vi "TestExec.Data Str to DataVariant.vi"(3 "error in":errorcluster, 4 "DataArray":string[](array[string]), 5 "DataStr":string) -> (0 "error out":errorcluster, 2 "Data":variant)   [LabVIEW 2017]
uses:
  Controls/TestExec.Result Cluster, Float.ctl
  Controls/TestExec.Comparison Enum.ctl
  Controls/TestExec.Result Cluster, Int.ctl
  Controls/TestExec.Result Cluster, Bool.ctl
  Controls/TestExec.Result Cluster, Str.ctl
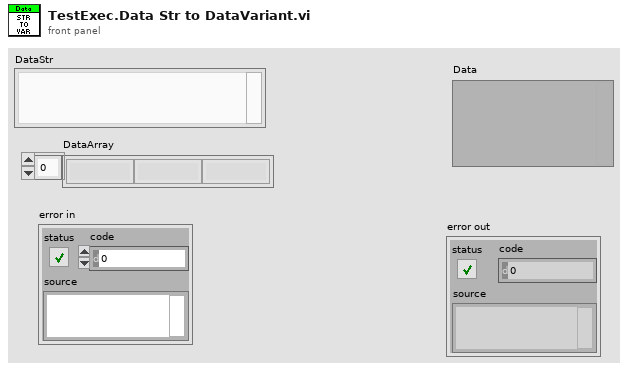
[diagram p1: front panel]
types:
  T1 = typedef "TestExec.Result Cluster, Str.ctl" = cluster{"Desc":string, "Value":string, "Units":string, "LimitName":string, "Comp1":T2, "Lim1":string, "Comp2":T2, "Lim2":string, "FailName":string, "FailCode":dbl, "FailDesc":string, "FailInfo":string}
  T2 = typedef "TestExec.Comparison Enum.ctl" = enum16{"N/A", "EQ", "NEQ", "LT", "LTE", "GT", "GTE"}
  T3 = typedef "TestExec.Result Cluster, Bool.ctl" = cluster{"Desc":string, "Value":bool, "Units":string, "LimitName":string, "Comp1":T2, "Lim1":bool, "FailName":string, "FailCode":dbl, "FailDesc":string, "FailInfo":string}
  T4 = typedef "TestExec.Result Cluster, Int.ctl" = cluster{"Desc":string, "Value":i32, "Units":string, "LimitName":string, "Comp1":T2, "Lim1":i32, "Comp2":T2, "Lim2":i32, "FailName":string, "FailCode":dbl, "FailDesc":string, "FailInfo":string}
  T5 = typedef "TestExec.Result Cluster, Float.ctl" = cluster{"Desc":string, "Value":dbl, "Units":string, "LimitName":string, "Comp1":T2, "Lim1":dbl, "Comp2":T2, "Lim2":dbl, "FailName":string, "FailCode":dbl, "FailDesc":string, "FailInfo":string}
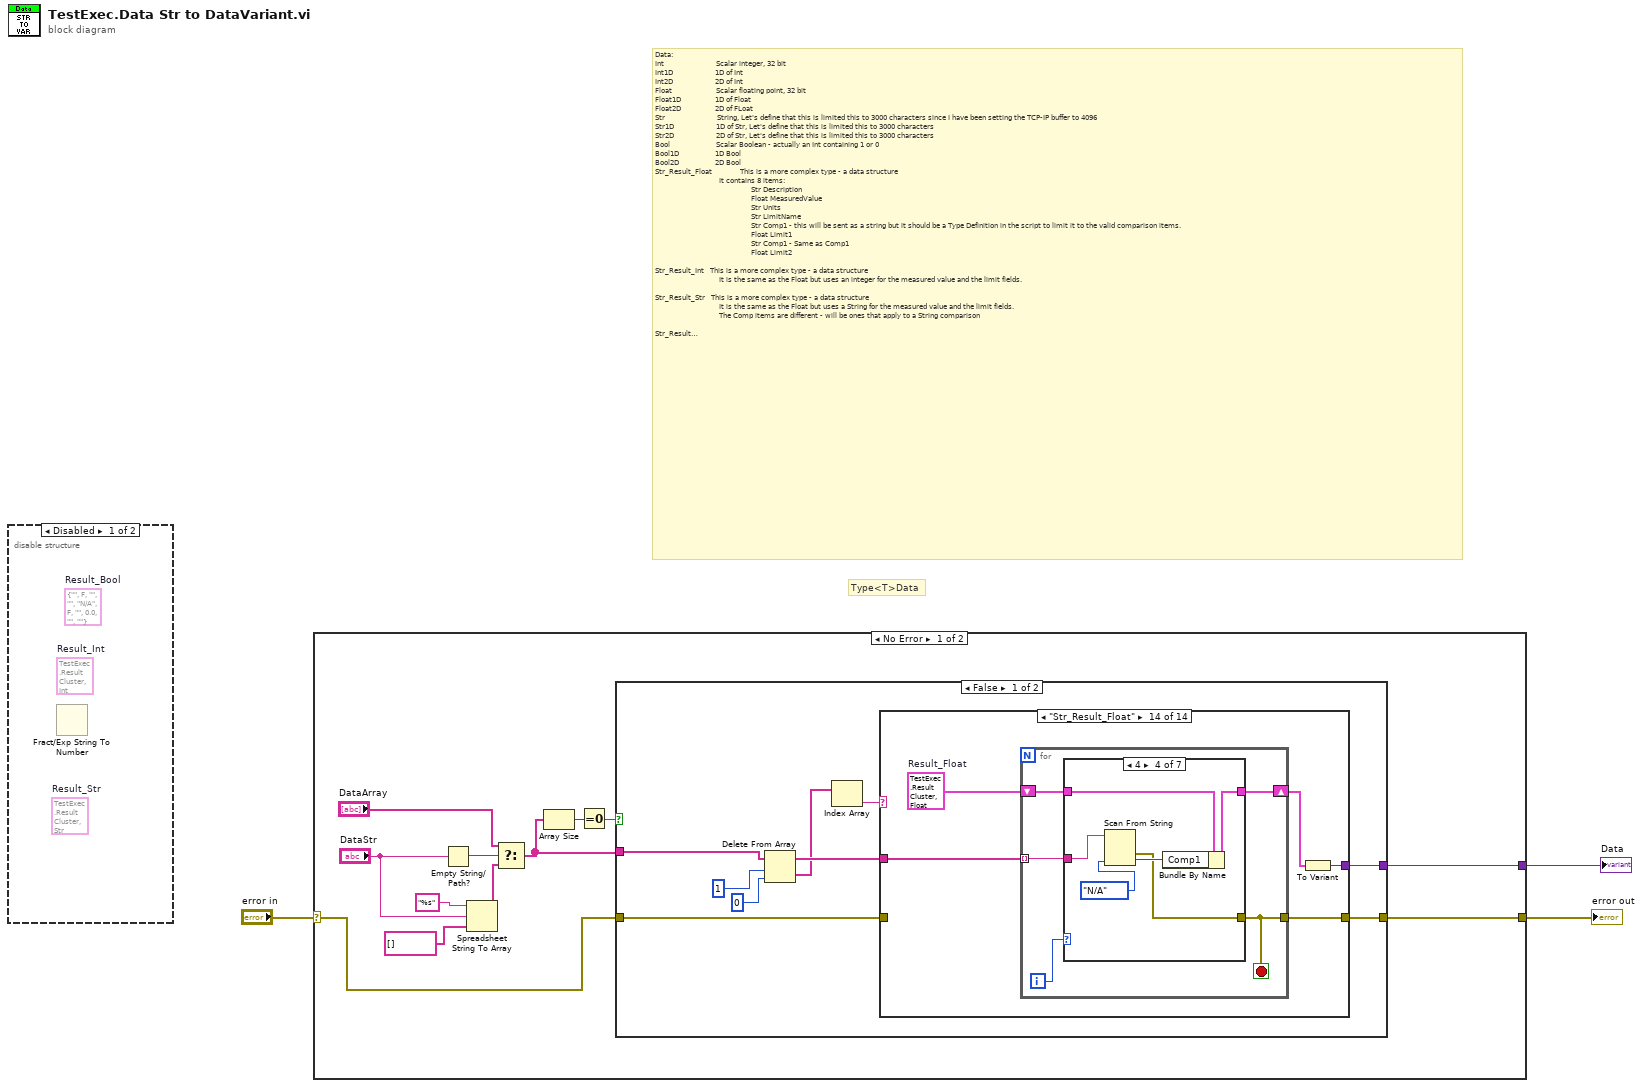
[diagram p0: block diagram]
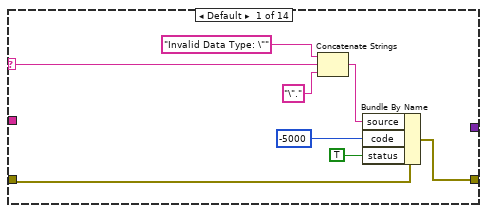
[diagram p3: hidden frame]
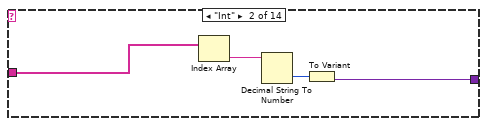
[diagram p4: hidden frame]
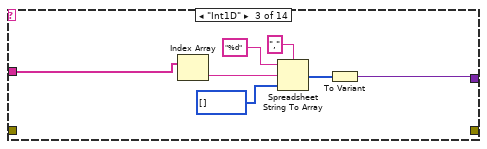
[diagram p5: hidden frame]
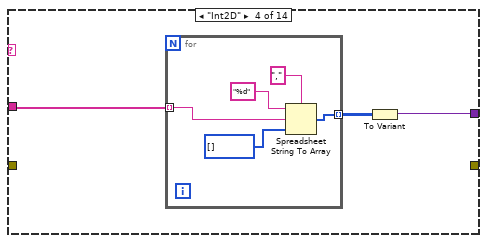
[diagram p6: hidden frame]
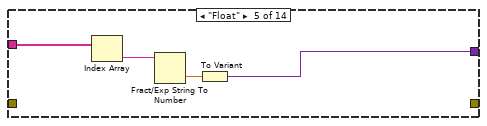
[diagram p7: hidden frame]
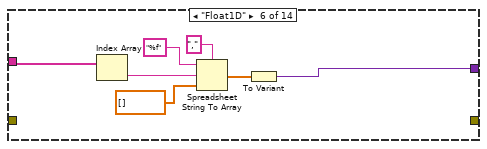
[diagram p8: hidden frame]
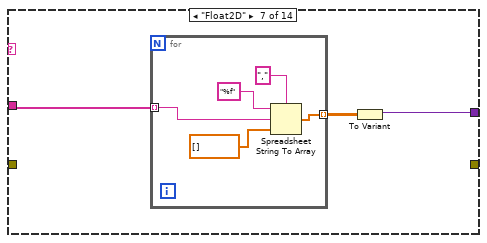
[diagram p9: hidden frame]
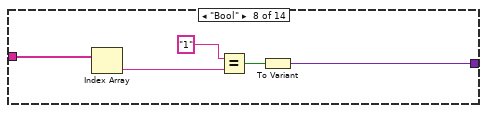
[diagram p10: hidden frame]
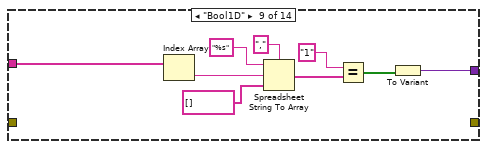
[diagram p11: hidden frame]
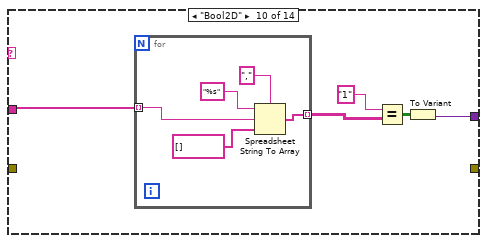
[diagram p12: hidden frame]
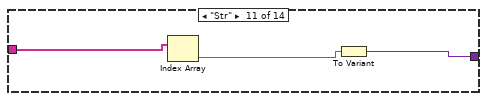
[diagram p13: hidden frame]
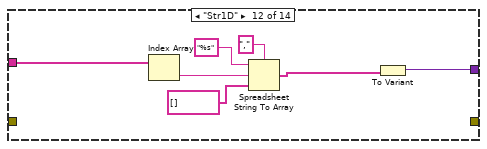
[diagram p14: hidden frame]
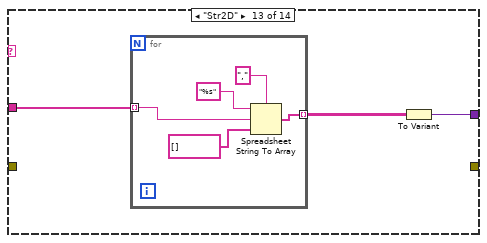
[diagram p15: hidden frame]
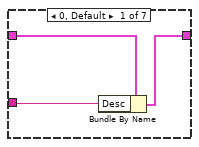
[diagram p16: hidden frame]
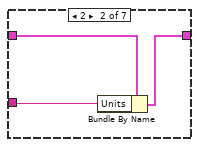
[diagram p17: hidden frame]
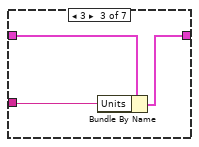
[diagram p18: hidden frame]
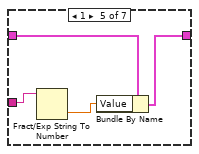
[diagram p19: hidden frame]
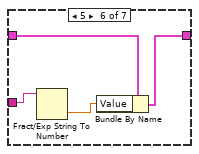
[diagram p20: hidden frame]
diagram:
  # "Data:\nInt                          Scalar integer, 32 bit\nInt1D                     1D of Int\nInt2D                     2D of Int\nFloat                      Scalar floating point, 32 bit\nFloat1D                 1D of Float\nFloat2D                 2D of FLoat\nStr                          String, Let's define that this is limited this to 3000 characters since I have been setting the TCP-IP buffer to 4096\nStr1D                     1D of Str, Let's define that this is limited this to 3000 characters\nStr2D                     2D of Str, Let's define that this is limited this to 3000 characters\nBool                       Scalar Boolean - actually an Int containing 1 or 0\nBool1D                  1D Bool\nBool2D                  2D Bool\nStr_Result_Float              This is a more complex type - a data structure\n                                It contains 8 items:\n                                                Str Description\n                                                Float MeasuredValue\n                                                Str Units\n                                                Str LimitName\n                                                Str Comp1 - this will be sent as a string but it should be a Type Definition in the script to limit it to the valid comparison items.\n                                                Float Limit1\n                                                Str Comp1 - Same as Comp1\n                                                Float Limit2\n \nStr_Result_Int   This is a more complex type - a data structure\n                                It is the same as the Float but uses an integer for the measured value and the limit fields.\n \nStr_Result_Str   This is a more complex type - a data structure\n                                It is the same as the Float but uses a String for the measured value and the limit fields.\n                                The Comp items are different - will be ones that apply to a String comparison\n \nStr_Result_Bool                This is a more complex type - a data structure\n                                It is the same as the Float but uses a Boolean for the measured value and the limit fields.\n                                The Comp items are different - will be ones that apply to a Bool comparison"
  # "Type<T>Data"
  n1 = disable-structure shown="Disabled" {
    frame Disabled {
      (unwired) T1 {"Desc"="", "Value"="", "Units"="", "LimitName"="", "Comp1"=enum."N/A", "Lim1"="", "Comp2"=enum."N/A", "Lim2"="", "FailName"="", "FailCode"=0.0, "FailDesc"="", "FailInfo"=""}  # Result_Str
      (unwired) T3 {"Desc"="", "Value"=FALSE, "Units"="", "LimitName"="", "Comp1"=enum."N/A", "Lim1"=FALSE, "FailName"="", "FailCode"=0.0, "FailDesc"="", "FailInfo"=""}  # Result_Bool
      (unwired) T4 {"Desc"="", "Value"=0, "Units"="", "LimitName"="", "Comp1"=enum."N/A", "Lim1"=0, "Comp2"=enum."N/A", "Lim2"=0, "FailName"="", "FailCode"=0.0, "FailDesc"="", "FailInfo"=""}  # Result_Int
      n2 = Fract/Exp String To Number() -> ()  [unwired: 4 in, 2 out]
    }
    frame Enabled {
    }
  }
  n3 = case shown="No Error" "error in" {
    selector: "error in" -> [w4 w153]
    tunnel: [w14 w153] -> w3
    tunnel: [w15 variant] -> w1
    frame No Error {
      n4 = Empty String/Path?(string/path="DataStr") -> (empty?=w9:bool)
      n5 = Spreadsheet String To Array(format string="%s", spreadsheet string="DataStr", array type (2D Dbl)=string[] []) -> (array=w11:string[])  [unwired: 1 in]
      n6 = Select(t="DataArray", s=w9, f=w11) -> (s? t:f=w6:string[])
      n7 = Array Size(array=w6) -> (size(s)=w13:i32)
      n8 = Equal To 0?(x=w13) -> (x = 0?=w5:bool)
      n9 = case shown="False" w5 {
        tunnel: [w23 variant] -> w15
        tunnel: w4 -> [w22 w150]
        tunnel: [w21 w150] -> w14
        tunnel: w6 -> [w16 _]
        frame False {
          n10 = Delete From Array(array=w16, length=1, index=0 ("length")) -> (deleted portion=w19:string[], array with subset deleted=w20:string[])
          n11 = Index Array(array=w19) -> (element=w24:string)  [unwired: 1 in]
          n12 = case shown="\"Str_Result_Float\"" w24 {
            selector: w24 -> [w25 _ _ _ _ _ _ _ _ _ _ _ _ _]
            tunnel: w20 -> [_ w33 w37 w44 w55 w57 w64 w75 w76 w85 w95 w98 w105 w116]
            tunnel: [_ w34 w38 w45 w54 w56 w63 w74 w77 w86 w96 w99 w106 w114] -> w23
            tunnel: w22 -> [w26 _ _ _ _ _ _ _ _ _ _ _ _ _]
            tunnel: [w27 _ _ _ _ _ _ _ _ _ _ _ _ w115] -> w21
            frame Default {
              n13 = Concatenate Strings("Invalid Data Type: \"", w25, "\".") -> (w28:string)
              n14 = Bundle By Name(cluster=w26, "source"=w28, "code"=-5000, "status"=TRUE) -> (w27:errorcluster)
            }
            frame "Int" {
              n15 = Index Array(array=w33) -> (element=w35:string)  [unwired: 1 in]
              n16 = Decimal String To Number(string=w35) -> (number=w36:i32)  [unwired: 2 in, 1 out]
              n17 = To Variant(anything=w36) -> (Variant=w34:variant)
            }
            frame "Int1D" {
              n18 = Index Array(array=w37) -> (element=w41:string)  [unwired: 1 in]
              n19 = Spreadsheet String To Array(delimiter (Tab)=",", format string="%d", spreadsheet string=w41, array type (2D Dbl)=i32[] []) -> (array=w42:i32[])
              n20 = To Variant(anything=w42) -> (Variant=w38:variant)
            }
            frame "Int2D" {
              n21 = for {
                tunnel: w44 -> [w48] mode=indexing
                tunnel: [w47] -> w46 mode=indexing
                n22 = Spreadsheet String To Array(delimiter (Tab)=",", format string="%d", spreadsheet string=w48, array type (2D Dbl)=i32[] []) -> (array=w47:i32[])
              }
              n23 = To Variant(anything=w46) -> (Variant=w45:variant)
            }
            frame "Float" {
              n24 = Index Array(array=w55) -> (element=w53:string)  [unwired: 1 in]
              n25 = Fract/Exp String To Number(string=w53) -> (number=w52:dbl)  [unwired: 3 in, 1 out]
              n26 = To Variant(anything=w52) -> (Variant=w54:variant)
            }
            frame "Float1D" {
              n27 = Index Array(array=w57) -> (element=w60:string)  [unwired: 1 in]
              n28 = Spreadsheet String To Array(delimiter (Tab)=",", format string="%f", spreadsheet string=w60, array type (2D Dbl)=dbl[] []) -> (array=w59:dbl[])
              n29 = To Variant(anything=w59) -> (Variant=w56:variant)
            }
            frame "Float2D" {
              n30 = for {
                tunnel: w64 -> [w67] mode=indexing
                tunnel: [w66] -> w65 mode=indexing
                n31 = Spreadsheet String To Array(delimiter (Tab)=",", format string="%f", spreadsheet string=w67, array type (2D Dbl)=dbl[] []) -> (array=w66:dbl[])
              }
              n32 = To Variant(anything=w65) -> (Variant=w63:variant)
            }
            frame "Bool" {
              n33 = Index Array(array=w75) -> (element=w71:string)  [unwired: 1 in]
              n34 = Equal?(x="1", y=w71) -> (x = y?=w73:bool)
              n35 = To Variant(anything=w73) -> (Variant=w74:variant)
            }
            frame "Bool1D" {
              n36 = Index Array(array=w76) -> (element=w80:string)  [unwired: 1 in]
              n37 = Spreadsheet String To Array(delimiter (Tab)=",", format string="%s", spreadsheet string=w80, array type (2D Dbl)=string[] []) -> (array=w83:string[])
              n38 = Equal?(x="1", y=w83) -> (x = y?=w84:bool[])
              n39 = To Variant(anything=w84) -> (Variant=w77:variant)
            }
            frame "Bool2D" {
              n40 = for {
                tunnel: w85 -> [w91] mode=indexing
                tunnel: [w90] -> w89 mode=indexing
                n41 = Spreadsheet String To Array(delimiter (Tab)=",", format string="%s", spreadsheet string=w91, array type (2D Dbl)=string[] []) -> (array=w90:string[])
              }
              n42 = Equal?(x="1", y=w89) -> (x = y?=w88:bool[][])
              n43 = To Variant(anything=w88) -> (Variant=w86:variant)
            }
            frame "Str" {
              n44 = Index Array(array=w95) -> (element=w97:string)  [unwired: 1 in]
              n45 = To Variant(anything=w97) -> (Variant=w96:variant)
            }
            frame "Str1D" {
              n46 = Index Array(array=w98) -> (element=w102:string)  [unwired: 1 in]
              n47 = Spreadsheet String To Array(delimiter (Tab)=",", format string="%s", spreadsheet string=w102, array type (2D Dbl)=string[] []) -> (array=w104:string[])
              n48 = To Variant(anything=w104) -> (Variant=w99:variant)
            }
            frame "Str2D" {
              n49 = for {
                tunnel: w105 -> [w109] mode=indexing
                tunnel: [w108] -> w107 mode=indexing
                n50 = Spreadsheet String To Array(delimiter (Tab)=",", format string="%s", spreadsheet string=w109, array type (2D Dbl)=string[] []) -> (array=w108:string[])
              }
              n51 = To Variant(anything=w107) -> (Variant=w106:variant)
            }
            frame "Str_Result_Float" {
              w117 = T5 {"Desc"="", "Value"=0.0, "Units"="", "LimitName"="", "Comp1"=enum."N/A", "Lim1"=0.0, "Comp2"=enum."N/A", "Lim2"=0.0, "FailName"="", "FailCode"=0.0, "FailDesc"="", "FailInfo"=""}  # Result_Float
              n52 = for {
                shift-right: [w121] -> w113
                shift-left: w117 -> [w122]
                tunnel: w116 -> [w119] mode=indexing
                tunnel: [w118] -> w115
                i -> [w120]
                stop <- w118 stop-if-true
                n53 = case shown="4" w120 {
                  tunnel: w122 -> [w125 w128 w131 w137 w141 w145 w149]
                  tunnel: [w124 w127 w130 w136 w140 w144 w148] -> w121
                  tunnel: w119 -> [w123 w126 w129 w133 w139 w143 w147]
                  tunnel: [_ _ _ w132 _ _ _] -> w118
                  frame 0, Default {
                    n54 = Bundle By Name(cluster=w125, "Desc"=w123) -> (w124:T5)
                  }
                  frame 2 {
                    n55 = Bundle By Name(cluster=w128, "Units"=w126) -> (w127:T5)
                  }
                  frame 3 {
                    n56 = Bundle By Name(cluster=w131, "Units"=w129) -> (w130:T5)
                  }
                  frame 4 {
                    n57 = Scan From String(input string=w133, default 1=TestExec.Comparison_Enum."N/A" ("Comp1")) -> (error out=w132:errorcluster, output 1=w135:T2)  [unwired: 3 in, 2 out]
                    n58 = Bundle By Name(cluster=w137, "Comp1"=w135) -> (w136:T5)
                  }
                  frame 1 {
                    n59 = Fract/Exp String To Number(string=w139) -> (number=w138:dbl)  [unwired: 3 in, 1 out]
                    n60 = Bundle By Name(cluster=w141, "Value"=w138) -> (w140:T5)
                  }
                  frame 5 {
                    n61 = Fract/Exp String To Number(string=w143) -> (number=w142:dbl)  [unwired: 3 in, 1 out]
                    n62 = Bundle By Name(cluster=w145, "Value"=w142) -> (w144:T5)
                  }
                  frame 7 {
                    n63 = Fract/Exp String To Number(string=w147) -> (number=w146:dbl)  [unwired: 3 in, 1 out]
                    n64 = Bundle By Name(cluster=w149, "Value"=w146) -> (w148:T5)
                  }
                }
              }
              n65 = To Variant(anything=w113) -> (Variant=w114:variant)
            }
          }
        }
        frame True {
          # "No Data\nOutput Void variant"
        }
      }
    }
    frame Error {
    }
  }
  "Data" <- w1
  "error out" <- w3
